vi "Main.vi"() -> ()   [LabVIEW 2013]
doc: "Use this template to build a simple state machine design pattern. Each state executes code and determines which state to transition to."
uses:
  controls/State.ctl
  controls/Data.ctl
  controls/Guess Status.ctl
panel:
  out "Match?":bool
  out "Random Number":i32
  out "Guess Status":T1=enum."Error"
  in  "Submit":bool
  in  "Guess":i32
  in  "Start":bool
  in  "Exit":bool
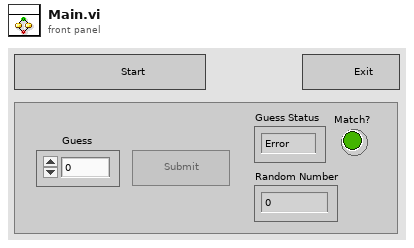
[diagram p1: front panel]
types:
  T1 = typedef "Guess Status.ctl" = enum16{"Equal", "Greater", "Less", "Error"}
  T2 = typedef "Data.ctl" = cluster{"Number of Guesses Limit":i32, "# Past Guesses":i32, "Number Range [Min,Max]":i32[], "Random Number":i32, "Guess":i32, "Guess Status":T1}
  T3 = typedef "State.ctl" = enum16{"Initialize", "Wait for Event", "Start", "Guess", "End Guessing", "Exit"}
  T4 = enum8{"Enabled", "Disabled", "Disabled and Grayed Out"}
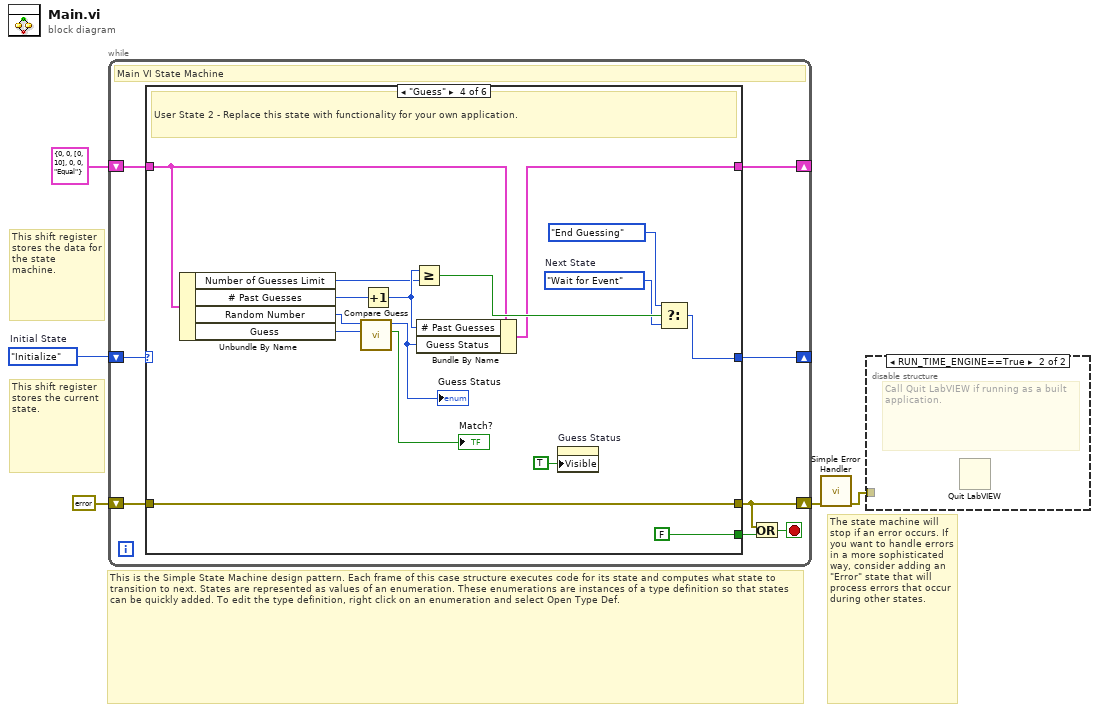
[diagram p0: block diagram]
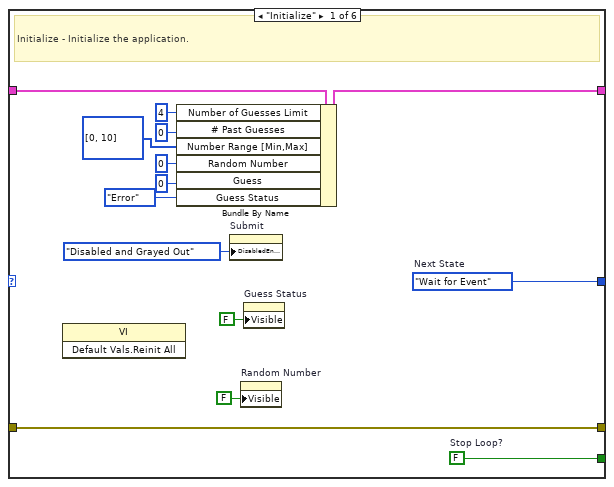
[diagram p3: hidden frame]
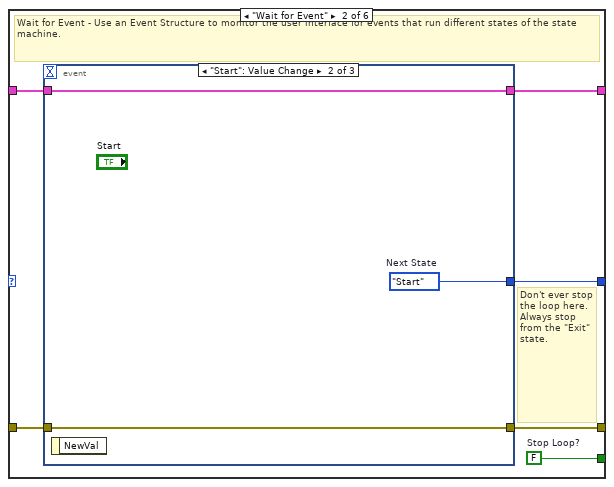
[diagram p4: hidden frame]
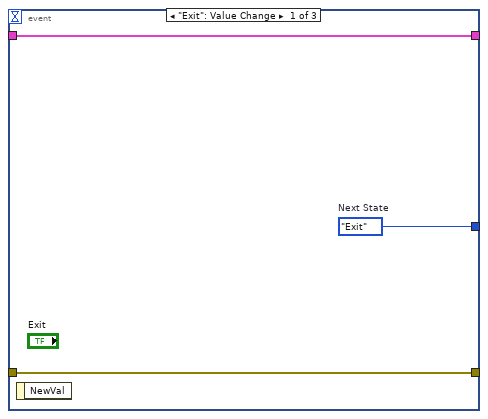
[diagram p5: hidden frame]
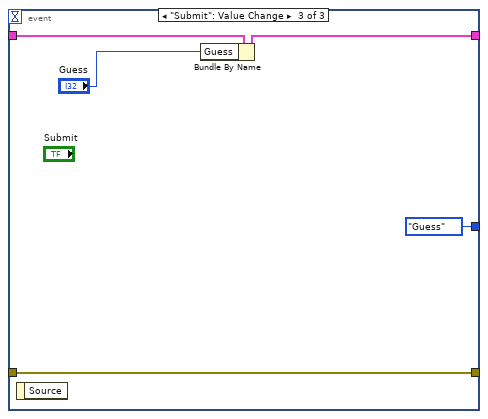
[diagram p6: hidden frame]
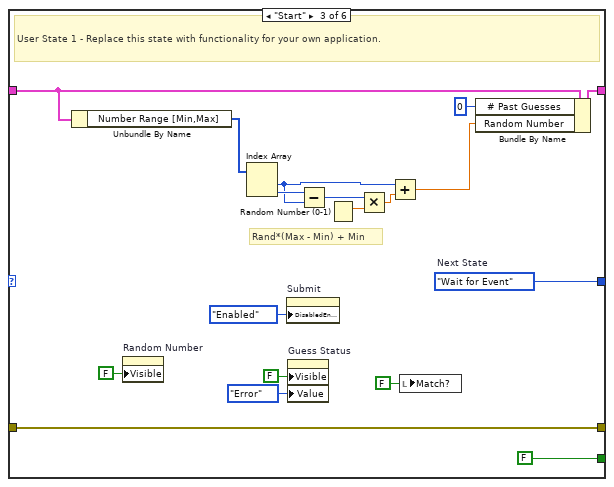
[diagram p7: hidden frame]
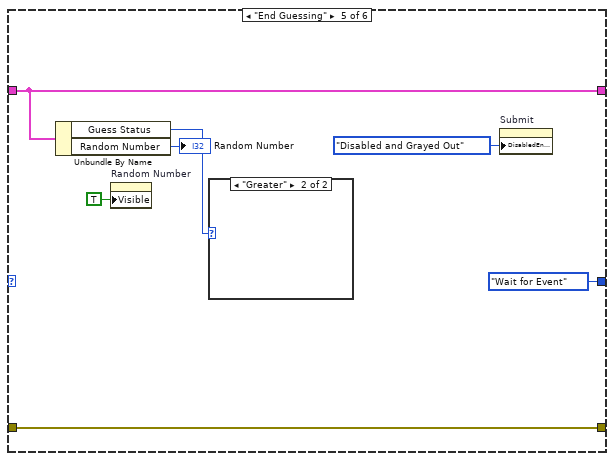
[diagram p8: hidden frame]
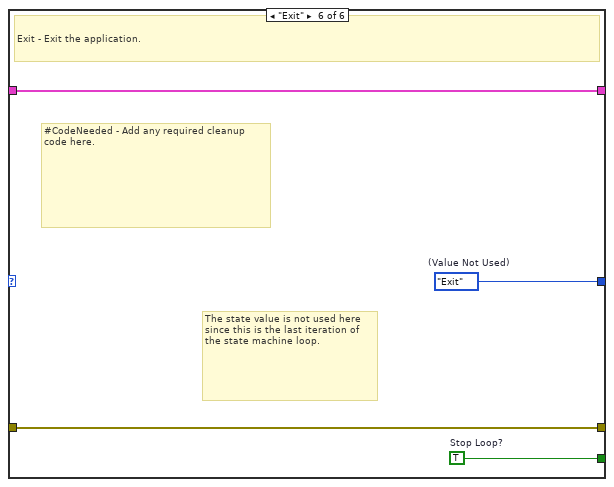
[diagram p10: hidden frame]
diagram:
  w5 = State."Initialize"  # Initial State
  # "The state machine will stop if an error occurs. If you want to handle errors in a more sophisticated way, consider adding an \"Error\" state that will process errors that occur during other states."
  # "This shift register stores the data for the state machine."
  # "This is the Simple State Machine design pattern. Each frame of this case structure executes code for its state and computes what state to transition to next. States are represented as values of an enumeration. These enumerations are instances of a type definition so that states can be quickly added. To edit the type definition, right click on an enumeration and select Open Type Def."
  # "This shift register stores the current state."
  n1 = while {
    shift-right: [w12] -> _
    shift-left: w5 -> [w13]
    shift-right: [w10] -> _
    shift-left: T2 {"Number of Guesses Limit"=0, "# Past Guesses"=0, "Number Range [Min,Max]"=[0, 10], "Random Number"=0, "Guess"=0, "Guess Status"=enum."Equal"} ("Data") -> [w11]
    shift-right: [w6] -> w2
    shift-left: errorcluster {"status"=FALSE, "code"=0, "source"=""} ("error constant") -> [w9]
    stop <- w7 stop-if-true
    # "Main VI State Machine"
    n2 = case shown="\"Guess\"" w13 {
      tunnel: [w27 w33 w62 w66 State."Wait for Event" ("(Value Not Used)") w89] -> w12
      tunnel: [w26 w32 FALSE ("Stop Loop?") FALSE ("Stop Loop?") _ w87] -> w8
      tunnel: w11 -> [w19 w31 w59 w67 w82 w88]
      tunnel: [w18 w30 w58 w65 w82 w88] -> w10
      tunnel: w9 -> [w25 w29 w60 w77 w85 w86]
      tunnel: [w25 w28 w60 w77 w85 w86] -> w6
      frame "Initialize" {
        w26 = FALSE  # Stop Loop?
        w27 = State."Wait for Event"  # Next State
        # "Initialize - Initialize the application."
        n3 = invoke class="VI" method="Default Vals.Reinit All"() -> ()  [unwired: 3 in, 3 out]
        n4 = Bundle By Name(cluster=w19, "Number of Guesses Limit"=4, "# Past Guesses"=0, "Number Range [Min,Max]"=i32[] [0, 10], "Random Number"=0, "Guess"=0, "Guess Status"=Guess_Status."Error") -> (w18:T2)
        n5 = property on="Submit" class="Bool"("DisabledEnum"=T4."Disabled and Grayed Out" ("Disabled")) -> ()  [unwired: 2 in, 2 out]
        n6 = property on="Random Number" class="DigNum (strict)"("Visible"=FALSE) -> ()  [unwired: 2 in, 2 out]
        n7 = property on="Guess Status" class="Enum (strict)"("Visible"=FALSE) -> ()  [unwired: 2 in, 2 out]
      }
      frame "Wait for Event" {
        w32 = FALSE  # Stop Loop?
        # "Don't ever stop the loop here. Always stop from the \"Exit\" state."
        # "Wait for Event - Use an Event Structure to monitor the user interface for events that run different states of the state machine."
        n8 = event shown="[1] \"Start\": Value Change" {
          selector: _ -> [_ _ _]
          dyn-events: _ -> [_ _ _]
          timeout: _ -> [_ _ _]
          tunnel: [w36 w39 State."Guess" ("Next State")] -> w33
          tunnel: w31 -> [w35 w37 w44]
          tunnel: [w35 w37 w41] -> w30
          tunnel: w29 -> [w34 w38 w43]
          tunnel: [w34 w38 w43] -> w28
          event "Exit": Value Change {
            w36 = State."Exit"  # Next State
            n9 = event-data() -> ()  [unwired: 1 in, 1 out]
          }
          event "Start": Value Change {
            w39 = State."Start"  # Next State
            n10 = event-data() -> ()  [unwired: 1 in, 1 out]
          }
          event "Submit": Value Change {
            n11 = event-data() -> ()  [unwired: 1 in, 1 out]
            n12 = Bundle By Name(cluster=w44, "Guess"="Guess") -> (w41:T2)
          }
        }
      }
      frame "Start" {
        w62 = State."Wait for Event"  # Next State
        # "Rand*(Max - Min) + Min"
        # "User State 1 - Replace this state with functionality for your own application."
        n13 = Unbundle By Name(w59) -> ("Number Range [Min,Max]"=w56:i32[])
        n14 = property on="Random Number" class="DigNum (strict)"("Visible"=FALSE) -> ()  [unwired: 2 in, 2 out]
        n15 = Index Array(array=w56) -> (element #1=w46:i32, element #2=w52:i32)  [unwired: 2 in]
        n16 = property on="Submit" class="Bool"("DisabledEnum"=T4."Enabled" ("Disabled")) -> ()  [unwired: 2 in, 2 out]
        n17 = property on="Guess Status" class="Enum (strict)"("Visible"=FALSE, "Value"=Guess_Status."Error" ("Guess Status")) -> ()  [unwired: 2 in, 2 out]
        n18 = Subtract(x=w52, y=w46) -> (x-y=w55:i32)
        n19 = Random Number (0-1)() -> (number: 0 to 1=w54:dbl)
        n20 = Multiply(x=w55, y=w54) -> (x*y=w53:dbl)
        n21 = Add(x=w46, y=w53) -> (x+y=w51:dbl)
        n22 = local write "Match?"(FALSE ("Match?")) -> ()
        n23 = Bundle By Name(cluster=w59, "# Past Guesses"=0, "Random Number"=w51) -> (w58:T2)
      }
      frame "Guess" {
        w68 = State."Wait for Event"  # Next State
        # "User State 2 - Replace this state with functionality for your own application."
        n24 = Unbundle By Name(w67) -> ("Number of Guesses Limit"=w70:i32, "# Past Guesses"=w69:i32, "Random Number"=w74:i32, "Guess"=w75:i32)
        n25 = call "Compare Guess.vi"("Guess"=w75, "Random Number"=w74) -> ("Match?"=→"Match?":bool, "Guess Status"=w76:T1)  [unwired: 8 in]
        "Guess Status" <- w76
        n26 = Increment(x=w69) -> (x+1=w73:i32)
        n27 = Greater Or Equal?(x=w73, y=w70) -> (x >= y?=w71:bool)
        n28 = Bundle By Name(cluster=w67, "# Past Guesses"=w73, "Guess Status"=w76) -> (w65:T2)
        n29 = property on="Guess Status" class="Enum (strict)"("Visible"=TRUE) -> ()  [unwired: 2 in, 2 out]
        n30 = Select(t=State."End Guessing", s=w71, f=w68) -> (s? t:f=w66:T3)
      }
      frame "End Guessing" {
        n31 = Unbundle By Name(w82) -> ("Guess Status"=w81:T1, "Random Number"=→"Random Number":i32)
        n32 = property on="Random Number" class="DigNum (strict)"("Visible"=TRUE) -> ()  [unwired: 2 in, 2 out]
        n33 = case shown="\"Greater\"" w81 {
          frame "Equal", Default {
          }
          frame "Greater" {
          }
        }
        n34 = property on="Submit" class="Bool"("DisabledEnum"=T4."Disabled and Grayed Out" ("Disabled")) -> ()  [unwired: 2 in, 2 out]
      }
      frame "Exit" {
        w87 = TRUE  # Stop Loop?
        w89 = State."Exit"  # (Value Not Used)
        # "#CodeNeeded - Add any required cleanup code here."
        # "The state value is not used here since this is the last iteration of the state machine loop."
        # "Exit - Exit the application."
      }
    }
    n35 = Or(x=w6, y=w8) -> (x .or. y?=w7:bool)
  }
  n36 = call <vilib>:"Simple Error Handler.vi"("error in (no error)"=w2) -> ("error out"=w1:errorcluster)  [unwired: 4 in, 4 out]
  n37 = disable-structure shown="RUN_TIME_ENGINE==True" {
    disable-tunnel: w1 -> [_ _]
    frame condition #0 (active) {
    }
    frame condition #1 {
      # "Call Quit LabVIEW if running as a built application."
      n38 = Quit LabVIEW() -> ()  [unwired: 1 in]
    }
  }
